vi "Fs_to_FilterDelay.vi"(11 "Fs":dbl) -> (3 "Total Filter Delay (samples)":dbl)   [LabVIEW 2016]
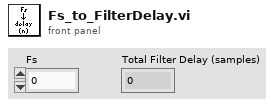
[diagram p1: front panel]
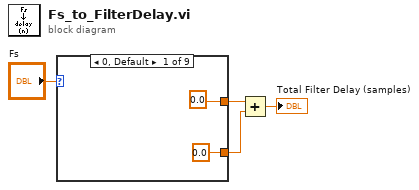
[diagram p0: block diagram]
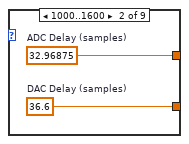
[diagram p2: hidden frame]
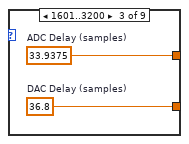
[diagram p3: hidden frame]
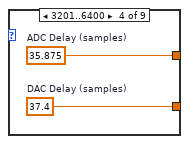
[diagram p4: hidden frame]
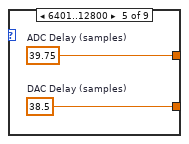
[diagram p5: hidden frame]
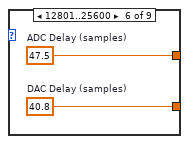
[diagram p6: hidden frame]
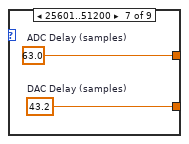
[diagram p7: hidden frame]
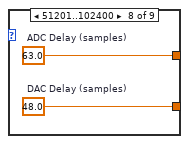
[diagram p8: hidden frame]
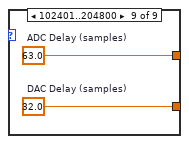
[diagram p9: hidden frame]
diagram:
  n1 = case shown="0, Default" "Fs" {
    tunnel: [0.0 ("ADC Delay (samples)") w8 w10 w12 w14 w16 w18 w20 w22] -> w3
    tunnel: [0.0 ("ADC Delay (samples)") w7 w9 w11 w13 w15 w17 w19 w21] -> w2
    frame 0, Default {
    }
    frame 1000..1600 {
      w7 = 36.6  # DAC Delay (samples)
      w8 = 32.96875  # ADC Delay (samples)
    }
    frame 1601..3200 {
      w9 = 36.8  # DAC Delay (samples)
      w10 = 33.9375  # ADC Delay (samples)
    }
    frame 3201..6400 {
      w11 = 37.4  # DAC Delay (samples)
      w12 = 35.875  # ADC Delay (samples)
    }
    frame 6401..12800 {
      w13 = 38.5  # DAC Delay (samples)
      w14 = 39.75  # ADC Delay (samples)
    }
    frame 12801..25600 {
      w15 = 40.8  # DAC Delay (samples)
      w16 = 47.5  # ADC Delay (samples)
    }
    frame 25601..51200 {
      w18 = 63.0  # ADC Delay (samples)
      w17 = 43.2  # DAC Delay (samples)
    }
    frame 51201..102400 {
      w20 = 63.0  # ADC Delay (samples)
      w19 = 48.0  # DAC Delay (samples)
    }
    frame 102401..204800 {
      w22 = 63.0  # ADC Delay (samples)
      w21 = 32.0  # DAC Delay (samples)
    }
  }
  n2 = Add(x=w3, y=w2) -> (x+y=→"Total Filter Delay (samples)":dbl)
